vi "Runmin1.vi"(8 "循环次数 i":i32, 9 "等待时间（毫秒）":u32=9, 10 "Queue1":T2, 11 "prodatascan":T1) -> (1 "runMin":dbl, 2 "AD":dbl)   [LabVIEW 2018]
uses:
  Initialize/CreateQueue/AllDataQueue.ctl
  Initialize/CreateQueue/SocketQueue.ctl
  Initialize/CreateQueue/LogDataQueue.ctl
  Initialize/CreateQueue/ProDataQueue.ctl
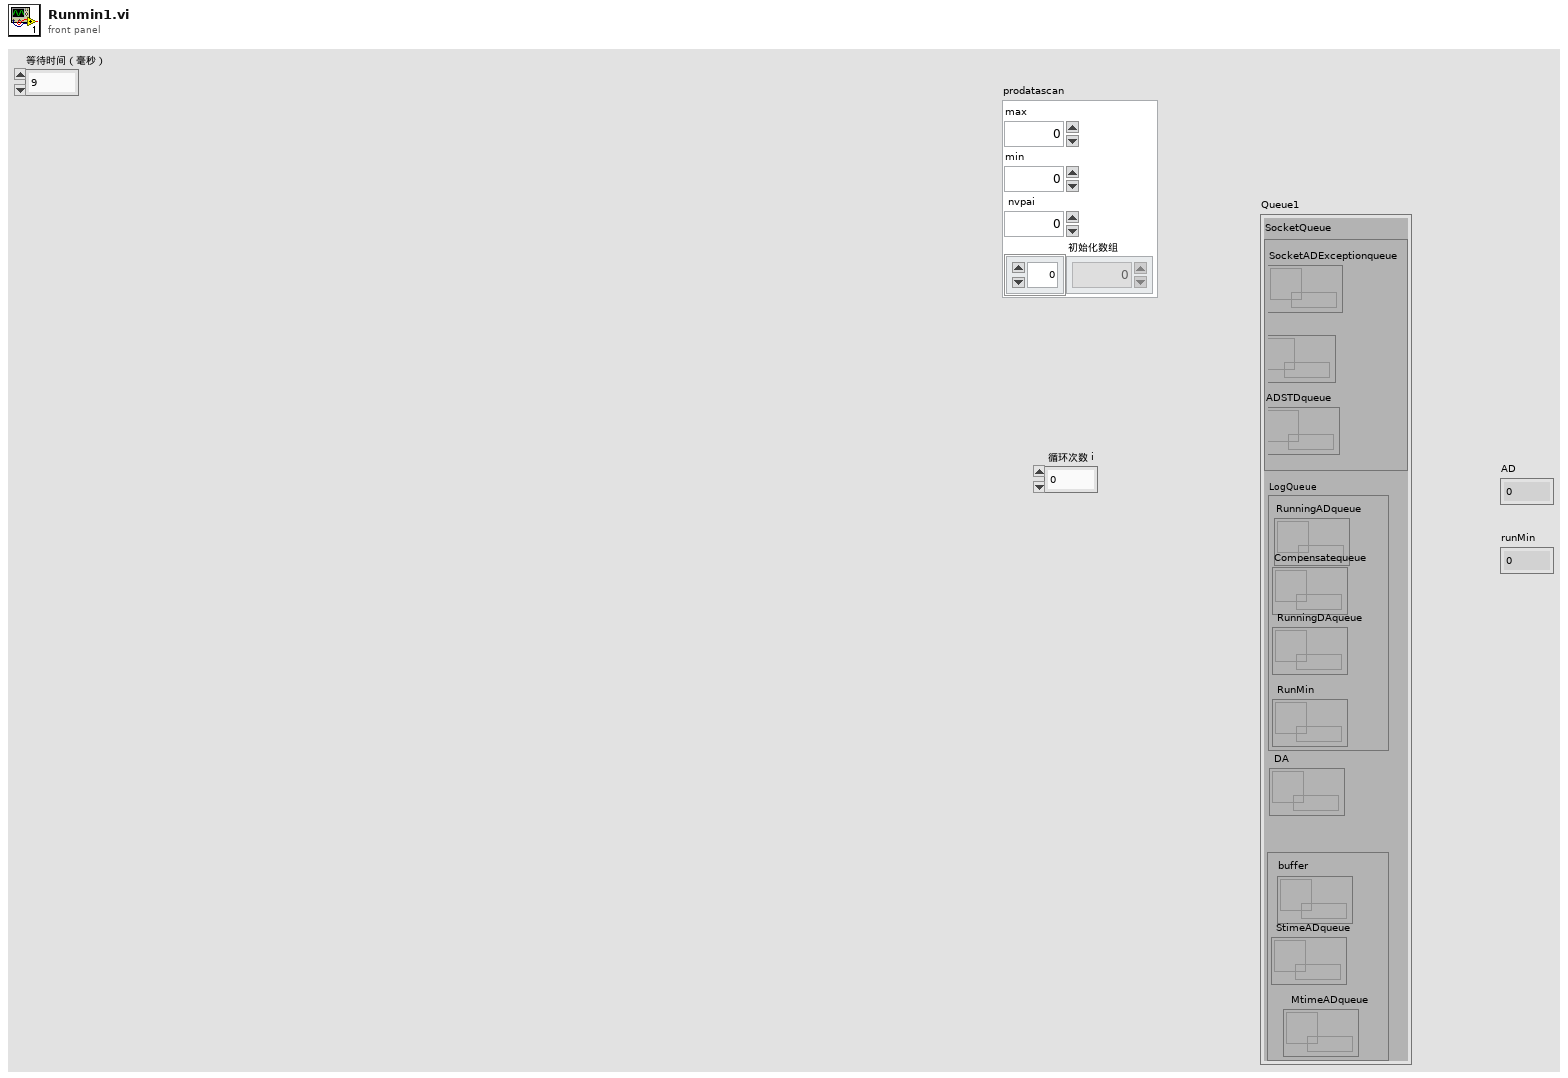
[diagram p1: front panel]
types:
  T1 = cluster{"max":dbl, "min":dbl, " nvpai":dbl, "初始化数组":dbl[]}
  T2 = typedef "AllDataQueue.ctl" = cluster{"SocketQueue":T3, "LogQueue":T4, " DA":refnum<queue>, "ProQueue":T5}
  T3 = typedef "SocketQueue.ctl" = cluster{"ADSTDqueue ":refnum<queue>, "SocketADExceptionqueue":refnum<queue>, "  SocketAD":refnum<queue>}
  T4 = typedef "LogDataQueue.ctl" = cluster{"RunningADqueue":refnum<queue>, "Compensatequeue":refnum<queue>, " RunningDAqueue":refnum<queue>, " RunMin":refnum<queue>}
  T5 = typedef "ProDataQueue.ctl" = cluster{"buffer ":refnum<queue>, " StimeADqueue":refnum<queue>, "  MtimeADqueue":refnum<queue>}
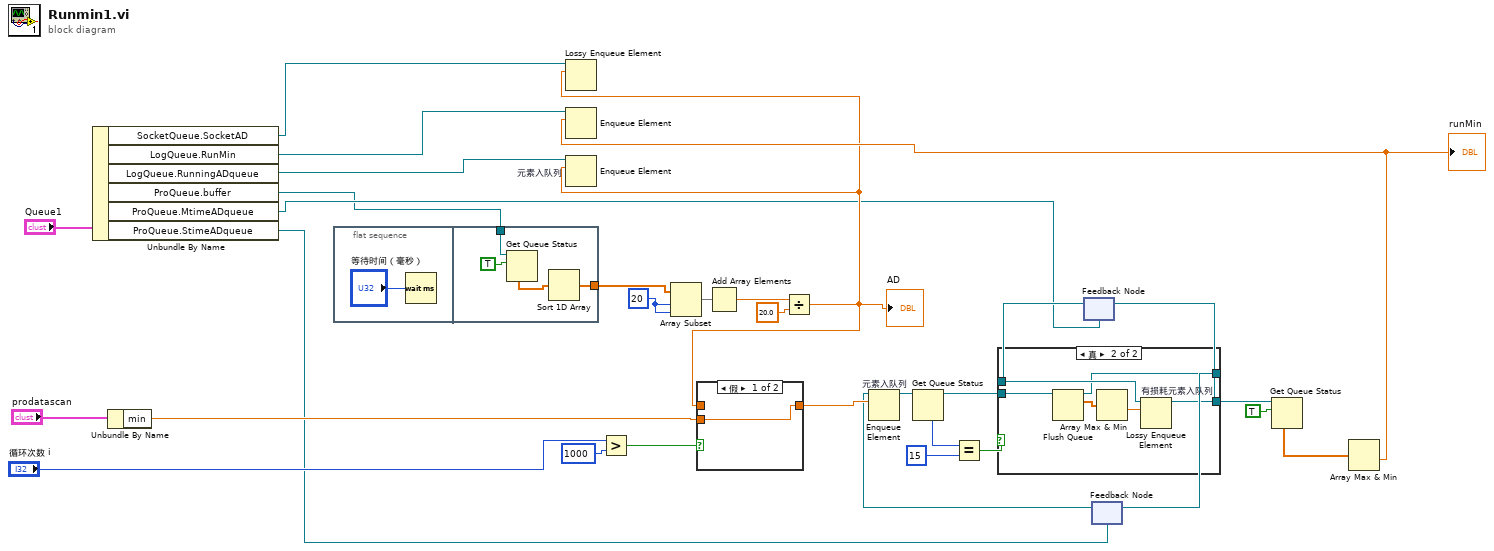
[diagram p0: block diagram]
diagram:
  w5 = 20 ("索引")
  n1 = Unbundle By Name("Queue1") -> ("SocketQueue.SocketAD"=w9:refnum<queue>, "LogQueue.RunMin"=w13:refnum<queue>, "LogQueue.RunningADqueue"=w12:refnum<queue>, "ProQueue.buffer"=w2:refnum<queue>, "ProQueue.MtimeADqueue"=w4:refnum<queue>, "ProQueue.StimeADqueue"=w3:refnum<queue>)
  n2 = Unbundle By Name("prodatascan") -> ("min"=w11:dbl)
  n3 = flat-sequence {
    tunnel: [w34] -> w1
    tunnel: w2 -> [w33]
    frame #0 {
      n4 = Wait (ms)(milliseconds to wait="等待时间（毫秒）") -> ()  [unwired: 1 out]
    }
    frame #1 {
      n5 = Get Queue Status(queue=w33, return elements? (F)=TRUE ("返回元素？(F)")) -> (elements=w35:dbl[])  [unwired: 1 in, 7 out]
      n6 = Sort 1D Array(array=w35) -> (sorted array=w34:dbl[])
    }
  }
  n7 = Greater?(x="循环次数 i", y=1000) -> (0:w25:bool)
  n8 = Array Subset(array=w1, index=w5, length=w5) -> (w28:dbl[])
  n9 = Add Array Elements(numeric array=w28) -> (sum=w29:dbl)
  n10 = Divide(x=w29, y=20.0) -> (x/y=w8:dbl)
  "AD" <- w8
  n11 = Lossy Enqueue Element(queue=w9, element=w8) -> ()  [unwired: 1 in, 4 out]
  n12 = Enqueue Element "元素入队列"(queue=w12, element=w8) -> ()  [unwired: 2 in, 3 out]
  n13 = case shown="假" w25 {
    tunnel: [w37 w38] -> w26
    tunnel: w8 -> [_ w38]
    tunnel: w11 -> [w37 _]
    frame False {
    }
    frame True {
    }
  }
  n14 = feedback #1(w4) -> (w21:refnum<queue>)
  n15 = feedback #2(w3) -> (w19:refnum<queue>)
  n16 = Enqueue Element "元素入队列"(queue=w19, element=w26) -> (queue out=w15:refnum<queue>)  [unwired: 2 in, 2 out]
  n17 = Get Queue Status(queue=w15) -> (queue out=w18:refnum<queue>, # elements in queue=w16:i32)  [unwired: 2 in, 6 out]
  n18 = Equal?(x=w16, y=15) -> (x = y?=w17:bool)
  n19 = case shown="真" w17 {
    tunnel: w18 -> [w40 w46]
    tunnel: w21 -> [w39 w43]
    tunnel: [w40 w42] -> w20
    tunnel: [w39 w41] -> w23
    frame False {
    }
    frame True {
      n20 = Flush Queue(queue=w46) -> (queue out=w42:refnum<queue>, remaining elements=w45:dbl[])  [unwired: 1 in, 1 out]
      n21 = Array Max & Min(array=w45) -> (min value=w44:dbl)  [unwired: 3 out]
      n22 = Lossy Enqueue Element "有损耗元素入队列"(queue=w43, element=w44) -> (queue out=w41:refnum<queue>)  [unwired: 1 in, 3 out]
    }
  }
  n23 = feedback-in #1(w23) -> ()
  n24 = feedback-in #2(w20) -> ()
  n25 = Get Queue Status(queue=w23, return elements? (F)=TRUE ("返回元素？(F)")) -> (elements=w24:dbl[])  [unwired: 1 in, 7 out]
  n26 = Array Max & Min(array=w24) -> (min value=w10:dbl)  [unwired: 3 out]
  "runMin" <- w10
  n27 = Enqueue Element(queue=w13, element=w10) -> ()  [unwired: 2 in, 3 out]
